vi "niRFSysCalReader Close.vi"(8 "error in":errorcluster, 11 "niRFSysCalReader Handle":T1) -> (0 "error out":errorcluster)   [LabVIEW 2016, in "niRFSysCalReader.lvlib"]
doc: "Releases the application memory reserved by the niRFSysCalReader Handle."
uses:
  niRFSysCalReader.lvlib
  INCLUDES/niRFSysCalReader Handle.ctl
  INCLUDES/niRFSysCalReader Core States.ctl
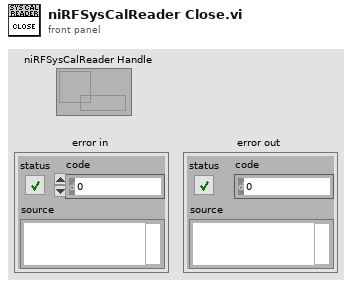
[diagram p1: front panel]
types:
  T1 = typedef "niRFSysCalReader.lvlib/niRFSysCalReader Handle.ctl" = refnum<data-value>
  T2 = typedef "niRFSysCalReader.lvlib/niRFSysCalReader Core States.ctl" = enum16{"Initialize", "Interpolator State", "Add CalData", "Get CalData", "Remove Pathloss", "Close"}
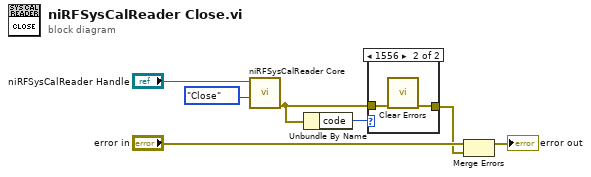
[diagram p0: block diagram]
diagram:
  n1 = call "niRFSysCalReader Core.vi"("niRFSysCalReader State"=niRFSysCalReader_Core_States."Close" ("Cal Storage"), "niRFSysCalReader Handle"="niRFSysCalReader Handle") -> ("error out"=w2:errorcluster)  [unwired: 7 in, 2 out]
  n2 = Unbundle By Name(w2) -> ("code"=w1:i32)
  n3 = case shown="1556" w1 {
    tunnel: [w8 w10] -> w4
    tunnel: w2 -> [w8 w9]
    frame Default {
    }
    frame 1556 {
      n4 = call <vilib>:"Clear Errors.vi"("error in (no error)"=w9) -> ("error out"=w10:errorcluster)  [unwired: 5 in, 1 out]
    }
  }
  n5 = Merge Errors("error in", w4) -> (→"error out":errorcluster)
